vi "Send Software Trigger.vi"(8 "error in (no error)":errorcluster, 11 "VISA resource name":refnum<visa-resource-name>) -> (0 "error out":errorcluster, 3 "VISA resource name out":refnum<visa-resource-name>)   [LabVIEW 2024]
doc: "A low-level VI that sends a software bus trigger to the instrument. You can use software bus triggers to trigger multipoint measurements. You must first set the <B>Trigger Source</B> control in the Configure Trigger VI to <B>Software (Bus)</B>. After each call to the<B> Initiate</B> VI, send a software bus trigger by calling this VI. When triggers are complete, call the <B>Fetch Multiple Points</B> VI. \n\n<B>Note:</B> Use this VI only with other low-level VIs. The high-level VIs automatically incorporate this functionality. \n\nThis VI does not check the instrument status. Typically, you call this VI only in a sequence of calls to other low-level instrument driver VIs. The sequence performs one operation. You use the low-level VIs to optimize one or more aspects of interaction with the instrument. If you want to check the instrument status, call the <B>Error Query</B> VI at the conclusion of the sequence."
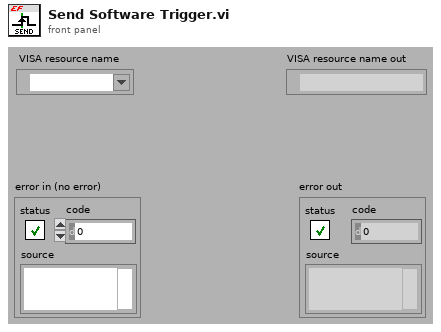
[diagram p1: front panel]
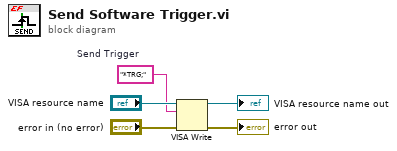
[diagram p0: block diagram]
diagram:
  w3 = "*TRG;"  # Send Trigger
  n1 = VISA Write(VISA resource name="VISA resource name", write buffer=w3, error in (no error)="error in (no error)") -> (VISA resource name out=→"VISA resource name out":refnum<visa-resource-name>, error out=→"error out":errorcluster)  [unwired: 1 out]
